vi "Mysql data reader 1D string.vi"(8 "error in (no error)":errorcluster, 11 ".NET Refnum in":refnum<k24>) -> (0 "error out":errorcluster, 3 "Array":string[](array[string]))   [LabVIEW 2020, in "mysql.lvlib" / "mysql.lvclass"]
uses:
  mysql.lvclass
  MySql.Data
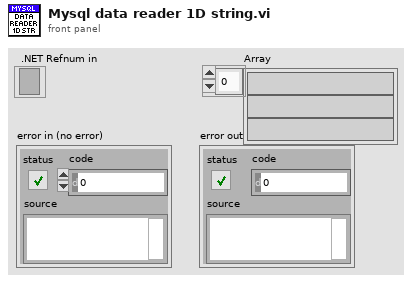
[diagram p1: front panel]
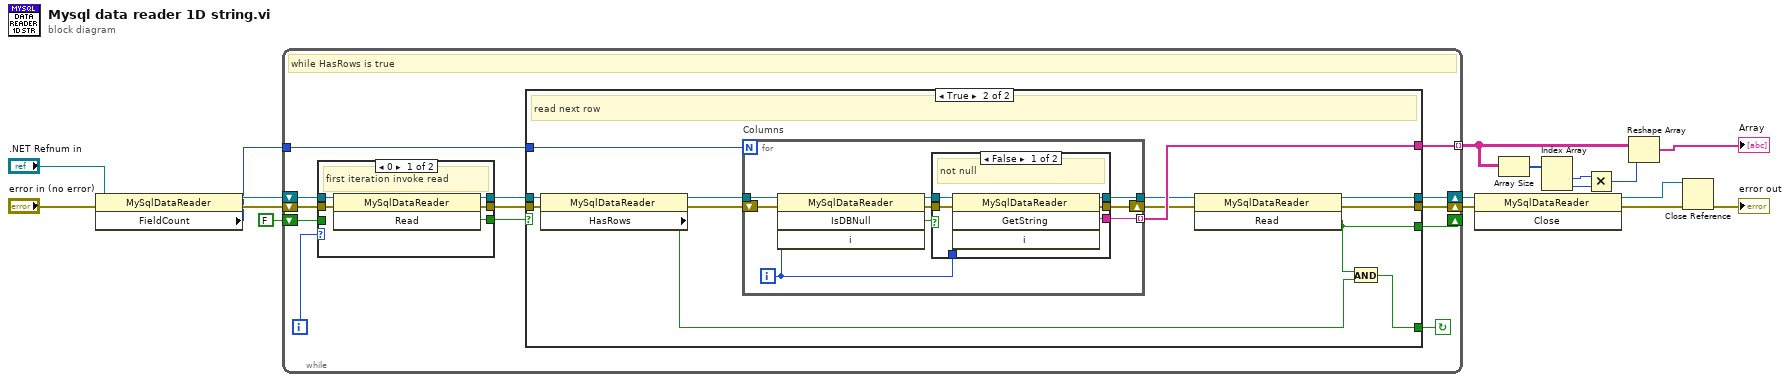
[diagram p0: block diagram]
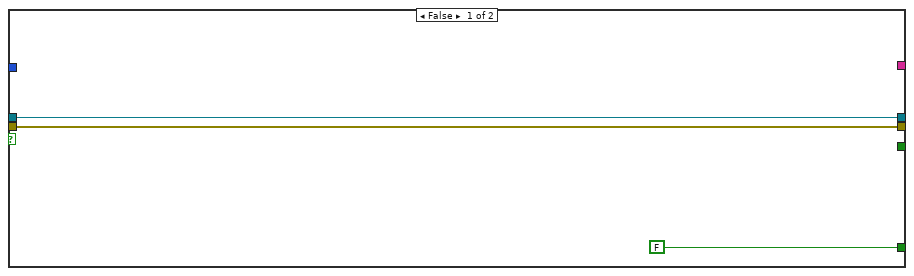
[diagram p3: hidden frame]
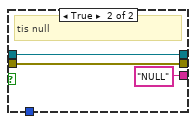
[diagram p4: hidden frame]
diagram:
  n1 = property class="MySqlDataReader"(reference=".NET Refnum in", error in="error in (no error)") -> (reference out=w13:refnum<k24>, error out=w12:errorcluster, "FieldCount"=w10:i32)
  n2 = while {
    tunnel: w10 -> [w30]
    tunnel: [w29] -> w3 mode=indexing
    shift-right: [w27] -> w15
    shift-left: w12 -> [w23]
    shift-right: [w28] -> w14
    shift-left: w13 -> [w24]
    shift-right: [w25] -> _
    shift-left: FALSE ("Read") -> [w22]
    i -> [w21]
    stop <- w26 continue-if-true
    # "while HasRows is true"
    n3 = case shown="0" w21 {
      tunnel: w23 -> [w35 w38]
      tunnel: [w34 w38] -> w20
      tunnel: w24 -> [w33 w36]
      tunnel: [w32 w37] -> w18
      tunnel: w22 -> [_ w37]
      tunnel: [w31 w36] -> w19
      frame 0 {
        # "first iteration invoke read"
        n4 = invoke class="MySqlDataReader" method="Read"(reference=w33, error in=w35) -> (reference out=w31:refnum<k24>, error out=w34:errorcluster, "Read"=w32:bool)  [unwired: 1 in]
      }
      frame 1.., Default {
        # "read after for other iterations"
      }
    }
    n5 = case shown="True" w18 {
      tunnel: w30 -> [_ w54]
      tunnel: [_ w53] -> w29
      tunnel: w20 -> [w40 w52]
      tunnel: w19 -> [w41 w51]
      tunnel: [w41 w47] -> w28
      tunnel: [w40 w45] -> w27
      tunnel: [FALSE ("HasRows") w43] -> w26
      tunnel: [_ w42] -> w25
      frame False {
      }
      frame True {
        # "read next row"
        n6 = property class="MySqlDataReader"(reference=w51, error in=w52) -> (reference out=w50:refnum<k24>, error out=w49:errorcluster, "HasRows"=w44:bool)
        n7 = for "Columns" {
          N: w54 -> [_]
          tunnel: w50 -> [w58]
          shift-right: [w63] -> w48
          shift-left: w49 -> [w59]
          tunnel: [w62] -> w53 mode=indexing
          tunnel: [w61] -> w46
          i -> [w60]
          n8 = invoke class="MySqlDataReader" method="IsDBNull"(reference=w58, error in=w59, "i"=w60) -> (reference out=w57:refnum<k24>, error out=w56:errorcluster, "IsDBNull"=w55:bool)  [unwired: 1 in, 1 out]
          n9 = case shown="False" w55 {
            tunnel: [w69 w71] -> w63
            tunnel: [w68 "NULL" ("GetString")] -> w62
            tunnel: [w67 w72] -> w61
            tunnel: w60 -> [w66 _]
            tunnel: w57 -> [w65 w72]
            tunnel: w56 -> [w64 w71]
            frame False {
              # "not null"
              n10 = invoke class="MySqlDataReader" method="GetString"(reference=w65, error in=w64, "i"=w66) -> (reference out=w67:refnum<k24>, error out=w69:errorcluster, "GetString"=w68:string)  [unwired: 1 in, 1 out]
            }
            frame True {
              # "tis null"
            }
          }
        }
        n11 = invoke class="MySqlDataReader" method="Read"(reference=w46, error in=w48) -> (reference out=w47:refnum<k24>, error out=w45:errorcluster, "Read"=w42:bool)  [unwired: 1 in]
        n12 = And(x=w42, y=w44) -> (x .and. y?=w43:bool)
      }
    }
  }
  n13 = invoke class="MySqlDataReader" method="Close"(reference=w14, error in=w15) -> (reference out=w17:refnum<k24>, error out=w16:errorcluster)  [unwired: 1 in, 1 out]
  n14 = Array Size(array=w3) -> (size(s)=w6:i32[])
  n15 = Index Array(array=w6) -> (element #1=w5:i32, element #2=w4:i32)  [unwired: 2 in]
  n16 = Multiply(x=w5, y=w4) -> (x*y=w1:i32)
  n17 = Reshape Array(w3, w1) -> (→"Array":string[])
  n18 = Close Reference(reference=w17, error in (no error)=w16) -> (error out=→"error out":errorcluster)
